vi "C to F .vi"() -> ()   [LabVIEW 2009]
panel:
  out "Farenheit":dbl(slide) scale=-200.0..200.0
  out "Waveform Chart":dbl(graph)
  in  "Celcius":dbl(slide) scale=-273.0..273.0
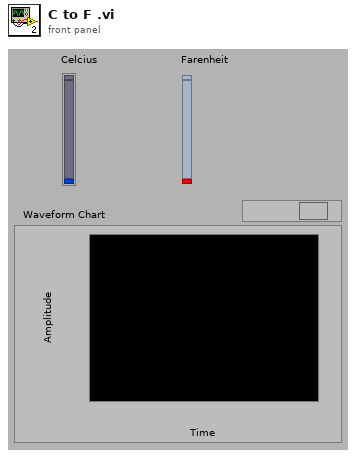
[diagram p1: front panel]
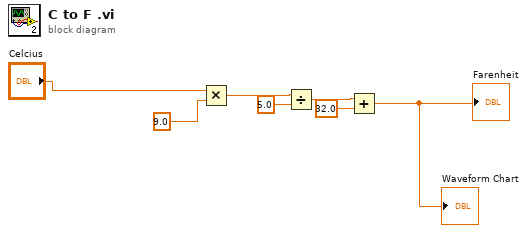
[diagram p0: block diagram]
diagram:
  n1 = Multiply(x="Celcius", y=9.0) -> (x*y=w6:dbl)
  n2 = Divide(x=w6, y=5.0) -> (x/y=w4:dbl)
  n3 = Add(x=w4, y=32.0) -> (x+y=→"Waveform Chart" →"Farenheit":dbl)
